vi "Gui_SetupSequence.vi"(7 "Variant For Path":variant, 8 "error in (no error)":errorcluster, 10 "Excit Table Variant":variant, 11 "Variant":variant) -> (0 "error out":errorcluster caption="sortie d'erreur", 2 "Excit Table Variant Output":variant, 3 "Variant Output":variant)   [LabVIEW 2018]
uses:
  controls/DATA_Inputs.ctl
  controls/PROCESSING_Inputs.ctl
  controls/TRAPPING_Inputs.ctl
  controls/SEQUENCE_Inputs.ctl
  controls/EXCIT_Inputs.ctl
  controls/TIMING_Inputs.ctl
panel:
  in  "SEQUENCE Inputs":T1={"EXCIT Inputs"={"Number of Excitations"=1, "Script Text"="", "Table of Waveforms"=[]}, "DATA Inputs"={"Record Length"=524000, "Sample Rate"=2000000.0, "Data Type"=0, "Vertical Range"=10.0, "Acquisition Duration"=262.0}, "TIMING Inputs"={"Number of Acquisitions "=1, "Number of Accumulations"=1, "Table of Waveforms"=[], "Script Text"=""}, "PROCESSING Inputs"={"Reference Mass"=300.0939, "Cyclotron Freq"=255.727, "Magnetron Freq"=0.001}, "TRAPPING Inputs"={"Number of Channels"=4, "Init Values"=[2.0, 9.0, 2.0, 9.0], "Opening Values"=[0.0, 0.0, 0.0, 0.0], "Trapping Values"=[2.0, 9.0, 2.0, 9.0], "Emptying Values"=[-10.0, -10.0, -10.0, -10.0], "Adiabatic ON"=FALSE, "Adiabatic Duration"=100, "Adiabatic Waveforms"=["Adiabatic_None_2_2_2000", "Adiabatic_Ramp_9_0_2000", "Adiabatic_None_2_2_2000", "Adiabatic_RC_9_0_2000"], "Ions Refill ON"=FALSE, "Number of Ions Refills"=1, "Trapping Delay"=400.0, "Trapping Duration"=300.0}} {"TRAPPING Inputs"."Trapping Duration" min=2.0; "TRAPPING Inputs"."Trapping Delay" min=2.0; "TRAPPING Inputs"."Number of Ions Refills" min=1 max=1000; "TRAPPING Inputs"."Trapping Values" min=-10.0 max=10.0; "TRAPPING Inputs"."Init Values" min=-10.0 max=10.0; "TRAPPING Inputs"."Emptying Values" min=-10.0 max=10.0; "TRAPPING Inputs"."Opening Values" min=-10.0 max=10.0; "PROCESSING Inputs"."Magnetron Freq" format="%.5g"; "PROCESSING Inputs"."Cyclotron Freq" format="%.5g"; "PROCESSING Inputs"."Reference Mass" format="%.5g"; "TIMING Inputs"."Number of Accumulations" min=0 max=50 step=1; "TIMING Inputs"."Number of Acquisitions" min=1 max=10 step=1; "DATA Inputs"."Vertical Range" items=["0.2"=0.2, "0.4"=0.4, "1"=1.0, "2"=2.0, "4"=4.0, "10"=10.0]; "DATA Inputs"."Data Type" items=["I16", "DBL"]; "DATA Inputs"."Sample Rate" items=["1 MHz"=1000000.0, "2 MHz"=2000000.0, "5 MHz"=5000000.0, "10 MHz"=10000000.0, "20 MHz"=20000000.0, "25 MHz"=25000000.0, "50 MHz"=50000000.0, "100 MHz"=100000000.0]; "EXCIT Inputs"."Number of Excitations" min=1 max=10}
  out "TRAPPING Inputs":T6={"Number of Channels"=4, "Init Values"=[2.0, 9.0, 2.0, 9.0], "Opening Values"=[0.0, 0.0, 0.0, 0.0], "Trapping Values"=[2.0, 9.0, 2.0, 9.0], "Emptying Values"=[-10.0, -10.0, -10.0, -10.0], "Adiabatic ON"=FALSE, "Adiabatic Duration"=100, "Adiabatic Waveforms"=["Adiabatic_None_2_2_2000", "Adiabatic_Ramp_9_0_2000", "Adiabatic_None_2_2_2000", "Adiabatic_RC_9_0_2000"], "Ions Refill ON"=FALSE, "Number of Ions Refills"=1, "Trapping Delay"=400.0, "Trapping Duration"=300.0} {"Trapping Duration" min=2.0; "Trapping Delay" min=2.0; "Number of Ions Refills" min=1 max=1000; "Trapping Values" min=-10.0 max=10.0; "Init Values" min=-10.0 max=10.0; "Emptying Values" min=-10.0 max=10.0; "Opening Values" min=-10.0 max=10.0}
  in  "Change Processing":bool
  out "PROCESSING Inputs":T5={"Reference Mass"=300.0939, "Cyclotron Freq"=255.727, "Magnetron Freq"=0.001} caption="DATA Inputs" {"Magnetron Freq" format="%.5g"; "Cyclotron Freq" format="%.5g"; "Reference Mass" format="%.5g"}
  in  "Change Trapping":bool
  in  "Change Data":bool
  out "DATA Inputs":T3={"Record Length"=100000, "Sample Rate"=10000000.0, "Data Type"=0, "Vertical Range"=10.0, "Acquisition Duration"=100000.0} {"Vertical Range" items=["0.2"=0.2, "0.4"=0.4, "1"=1.0, "2"=2.0, "4"=4.0, "10"=10.0]; "Data Type" items=["I16", "DBL"]; "Sample Rate" items=["1 MHz"=1000000.0, "2 MHz"=2000000.0, "5 MHz"=5000000.0, "10 MHz"=10000000.0, "20 MHz"=20000000.0, "25 MHz"=25000000.0, "50 MHz"=50000000.0, "100 MHz"=100000000.0]}
  in  "Change Excitation":bool
  out "Excitation Script":string
  out "Timing Script":string
  in  "Change Timing":bool
  in  "Exit":bool
  # "GO_out"
  # "Gout"
  # "GI_in"
  # "Gin"
  # "GO_out"
  # "Gout"
  # "GI_in"
  # "Gin"
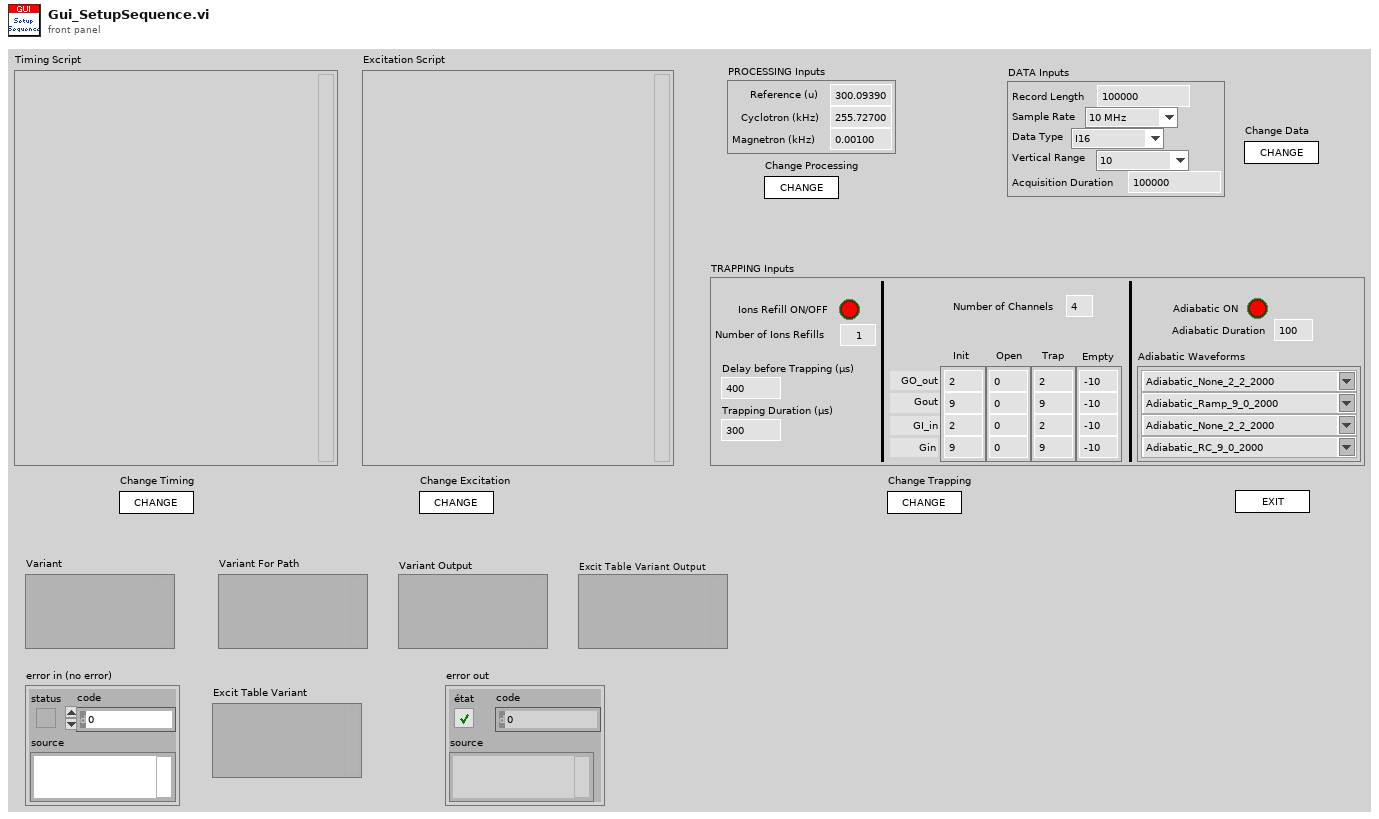
[diagram p1: front panel]
types:
  T1 = typedef "SEQUENCE_Inputs.ctl" = cluster{"EXCIT Inputs":T2, "DATA Inputs":T3, "TIMING Inputs":T4, "PROCESSING Inputs":T5, "TRAPPING Inputs":T6}
  T2 = typedef "EXCIT_Inputs.ctl" = cluster{"Number of Excitations":i32, "Script Text":string, "Table of Waveforms":string[]}
  T3 = typedef "DATA_Inputs.ctl" = cluster{"Record Length":i32, "Sample Rate":dbl, "Data Type":u8, "Vertical Range":dbl, "Acquisition Duration":dbl}
  T4 = typedef "TIMING_Inputs.ctl" = cluster{"Number of Acquisitions ":i16, "Number of Accumulations":i16, "Table of Waveforms":string[], "Script Text":string}
  T5 = typedef "PROCESSING_Inputs.ctl" = cluster{"Reference Mass":dbl, "Cyclotron Freq":dbl, "Magnetron Freq":dbl}
  T6 = typedef "TRAPPING_Inputs.ctl" = cluster{"Number of Channels":i32, "Init Values":dbl[], "Opening Values":dbl[], "Trapping Values":dbl[], "Emptying Values":dbl[], "Adiabatic ON":bool, "Adiabatic Duration":i32, "Adiabatic Waveforms":string[], "Ions Refill ON":bool, "Number of Ions Refills":i32, "Trapping Delay":dbl, "Trapping Duration":dbl}
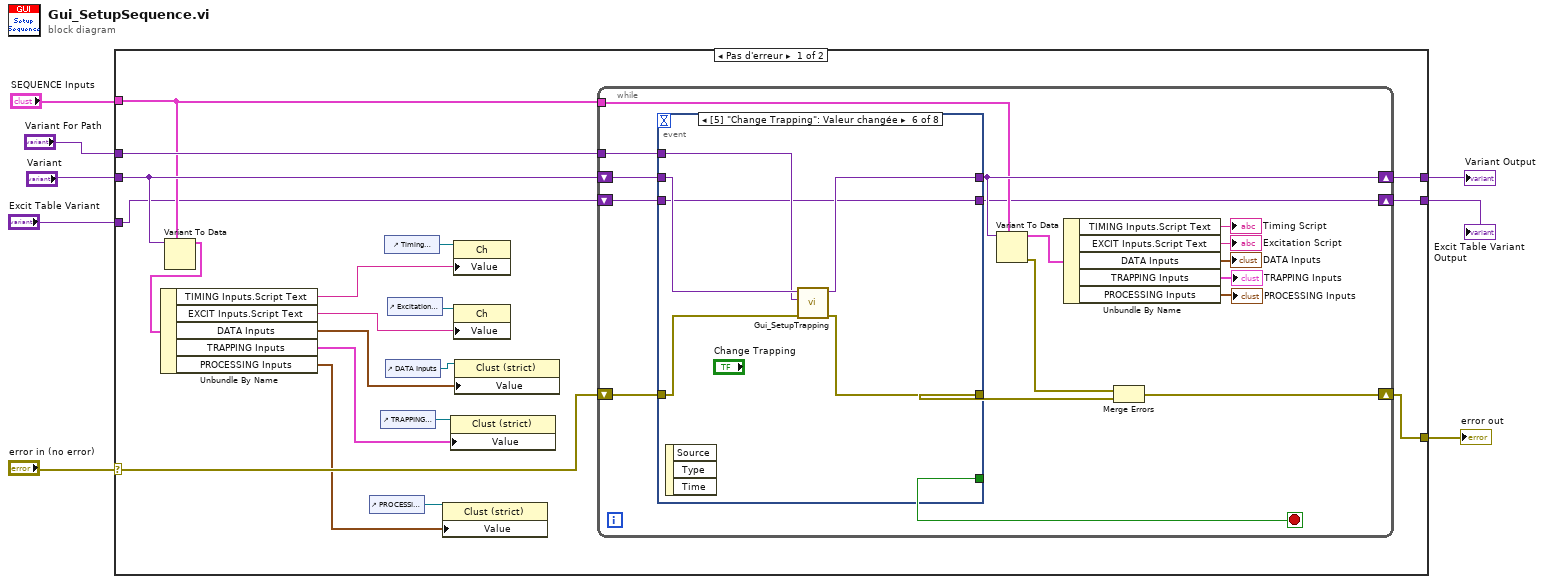
[diagram p0: block diagram]
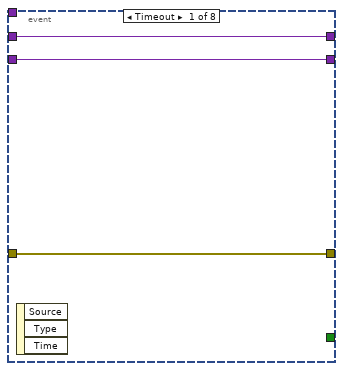
[diagram p2: hidden frame]
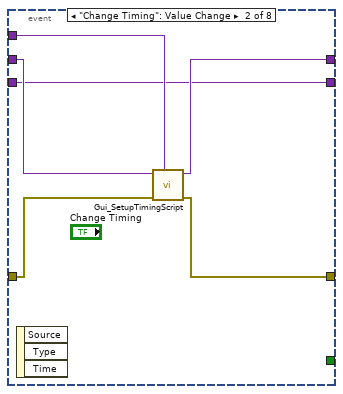
[diagram p3: hidden frame]
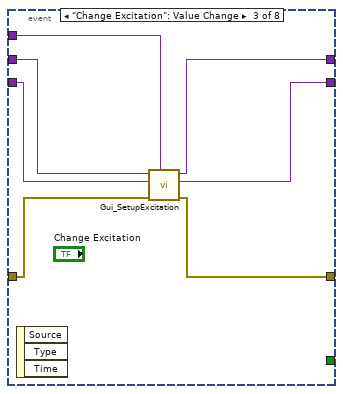
[diagram p4: hidden frame]
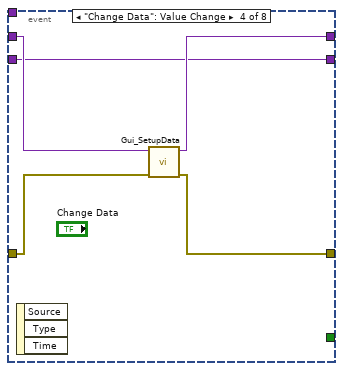
[diagram p5: hidden frame]
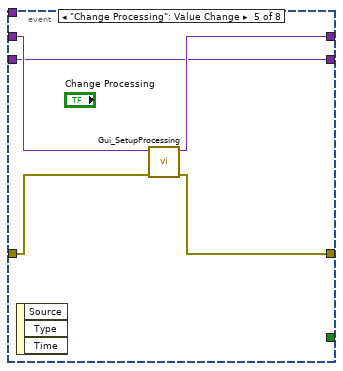
[diagram p6: hidden frame]
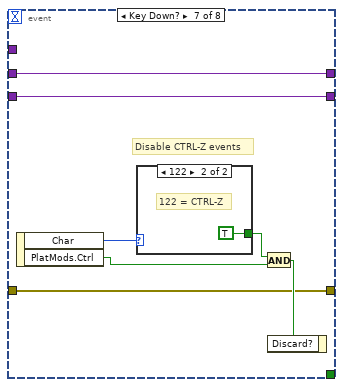
[diagram p7: hidden frame]
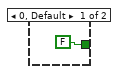
[diagram p8: hidden frame]
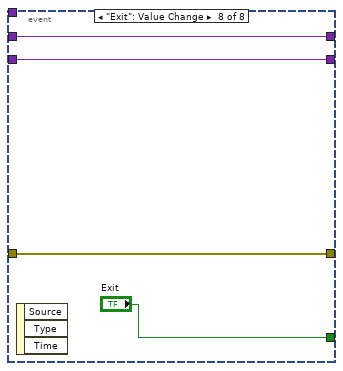
[diagram p9: hidden frame]
diagram:
  n1 = case shown="Pas d'erreur" "error in (no error)" {
    selector: "error in (no error)" -> [w25 w92]
    tunnel: "Variant" -> [w23 w91]
    tunnel: [w24 w92] -> w6
    tunnel: "Variant For Path" -> [w27 _]
    tunnel: [w26 w91] -> w4
    tunnel: "SEQUENCE Inputs" -> [w15 _]
    tunnel: "Excit Table Variant" -> [w12 w90]
    tunnel: [w11 w90] -> w2
    frame No Error {
      n2 = Variant To Data(type=w15, Variant=w23) -> (data=w16:T1)  [unwired: 1 in, 1 out]
      n3 = Unbundle By Name(w16) -> ("TIMING Inputs.Script Text"=w21:string, "EXCIT Inputs.Script Text"=w19:string, "DATA Inputs"=w18:T3, "TRAPPING Inputs"=w10:T6, "PROCESSING Inputs"=w13:T5)
      n4 = control-ref of="PROCESSING Inputs"() -> (w14:refnum<vi>)
      n5 = control-ref of="TRAPPING Inputs"() -> (w9:refnum<vi>)
      n6 = control-ref of="Timing Script"() -> (w22:refnum<vi>)
      n7 = control-ref of="DATA Inputs"() -> (w17:refnum<vi>)
      n8 = control-ref of="Excitation Script"() -> (w20:refnum<vi>)
      n9 = property class="Clust (strict)"(reference=w14, "Value"=w13) -> ()  [unwired: 1 in, 2 out]
      n10 = property class="Clust (strict)"(reference=w9, "Value"=w10) -> ()  [unwired: 1 in, 2 out]
      n11 = property class="Ch"(reference=w22, "Value"=w21) -> ()  [unwired: 1 in, 2 out]
      n12 = property class="Ch"(reference=w20, "Value"=w19) -> ()  [unwired: 1 in, 2 out]
      n13 = property class="Clust (strict)"(reference=w17, "Value"=w18) -> ()  [unwired: 1 in, 2 out]
      n14 = while {
        tunnel: w27 -> [w44]
        shift-right: [w40] -> w26
        shift-left: w23 -> [w43]
        shift-right: [w36] -> w24
        shift-left: w25 -> [w42]
        tunnel: w15 -> [w32]
        shift-right: [w30] -> w11
        shift-left: w12 -> [w29]
        stop <- w41 stop-if-true
        n15 = event shown="[5] \"Change Trapping\": Valeur changée" {
          selector: _ -> [_ _ _ _ _ _ _ _]
          dyn-events: _ -> [_ _ _ _ _ _ _ _]
          timeout: _ -> [_ _ _ _ _ _ _ _]
          tunnel: w44 -> [_ w52 w58 _ _ w72 _ _]
          tunnel: w43 -> [w46 w53 w57 w62 w67 w73 w78 w88]
          tunnel: w42 -> [w47 w51 w60 w65 w70 w76 w77 w87]
          tunnel: [w47 w50 w59 w63 w68 w74 w77 w87] -> w37
          tunnel: [w46 w49 w54 w64 w69 w75 w78 w88] -> w40
          tunnel: [_ _ _ _ _ _ _ "Exit"] -> w41
          tunnel: w29 -> [w45 w48 w56 w61 w66 w71 w79 w86]
          tunnel: [w45 w48 w55 w61 w66 w71 w79 w86] -> w30
          event Timeout {
            n16 = event-data() -> ()  [unwired: 1 in, 3 out]
          }
          event "Change Timing": Value Change {
            n17 = event-data() -> ()  [unwired: 1 in, 3 out]
            n18 = call "Gui_SetupTimingScript.vi"("Variant For Path"=w52, "error in (no error)"=w51, "Variant"=w53) -> ("error out"=w50:errorcluster, "Variant Output"=w49:variant)  [unwired: 7 in]
          }
          event "Change Excitation": Value Change {
            n19 = event-data() -> ()  [unwired: 1 in, 3 out]
            n20 = call "Gui_SetupExcitation.vi"("Variant For Path"=w58, "error in (no error)"=w60, "Excit Table Variant"=w56, "Variant"=w57) -> ("error out"=w59:errorcluster, "Excit Table Variant Output"=w55:variant, "Variant Output"=w54:variant)  [unwired: 5 in]
          }
          event "Change Data": Value Change {
            n21 = event-data() -> ()  [unwired: 1 in, 3 out]
            n22 = call "Gui_SetupData.vi"("error in (no error)"=w65, "Variant"=w62) -> ("error out"=w63:errorcluster, "Variant out"=w64:variant)  [unwired: 8 in]
          }
          event "Change Processing": Value Change {
            n23 = event-data() -> ()  [unwired: 1 in, 3 out]
            n24 = call "Gui_SetupProcessing.vi"("error in (no error)"=w70, "Variant"=w67) -> ("error out"=w68:errorcluster, "Variant out"=w69:variant)  [unwired: 8 in]
          }
          event "Change Trapping": Value Change {
            n25 = event-data() -> ()  [unwired: 1 in, 3 out]
            n26 = call "Gui_SetupTrapping.vi"("error in (no error)"=w76, "Variant for Path"=w72, "Variant"=w73) -> ("error out"=w74:errorcluster, "Variant out"=w75:variant)  [unwired: 7 in]
          }
          event Key Down? {
            # "Disable CTRL-Z events"
            n27 = event-data() -> ("Char"=w82:i16, "PlatMods.Ctrl"=w81:bool)  [unwired: 1 in]
            n28 = case shown="122" w82 {
              tunnel: [FALSE TRUE] -> w83
              frame 0, Default {
              }
              frame 122 {
                # "122 = CTRL-Z"
              }
            }
            n29 = And(x=w83, y=w81) -> (x .and. y?=w80:bool)
            n30 = event-data("Discard?"=w80) -> ()  [unwired: 1 in, 1 out]
          }
          event "Exit": Value Change {
            n31 = event-data() -> ()  [unwired: 1 in, 3 out]
          }
        }
        n32 = Variant To Data(type=w32, Variant=w40) -> (data=w39:T1, error out=w38:errorcluster)  [unwired: 1 in]
        n33 = Unbundle By Name(w39) -> ("TIMING Inputs.Script Text"=→"Timing Script":string, "EXCIT Inputs.Script Text"=→"Excitation Script":string, "DATA Inputs"=→"DATA Inputs":T3, "TRAPPING Inputs"=→"TRAPPING Inputs":T6, "PROCESSING Inputs"=→"PROCESSING Inputs":T5)
        n34 = Merge Errors(w38, w37) -> (w36:errorcluster)
      }
    }
    frame Error {
    }
  }
  "error out" <- w6
  "Variant Output" <- w4
  "Excit Table Variant Output" <- w2
